vi "Outputs.vi"(0 "STEP in":T1, 5 "CORE":refnum<queue>, 7 "Mapping Buss":T9, 9 "STEP State":T8, 11 "error in (no error)":errorcluster, 12 "Variables State in":T6, 13 "HW CTRL Data":T7) -> (4 "STEP out":T1, 15 "error out":errorcluster)   [LabVIEW 2014, in "SeqLoop.lvlib"]
doc: "Gestiona las Salidas Digitales."
uses:
  TypeDefs/HW InOut MAP.ctl
  TypeDefs/STEP State.ctl
  APIs/Message Queue/Message Cluster.ctl
  TypeDefs/HW CTRL Data.ctl
  TypeDefs/HW Variables State.ctl
  TypeDefs/STEP.ctl
  TypeDefs/LogicParsedExpression.ctl
  Mimico Display/TypeDefs/Mimic Data.ctl
  Mimico Display/TypeDefs/BG Image.ctl
  Mimico Display/TypeDefs/mObject.ctl
  DO Monitoring Global Variables.vi
  APIs/Message Queue/Enqueue Message (Single).vi
  SeqLoop.lvlib
  APIs/Message Queue/WINFAS 2 Message Queue.lvlib
  Mimico Display/Mimico Display.lvlib
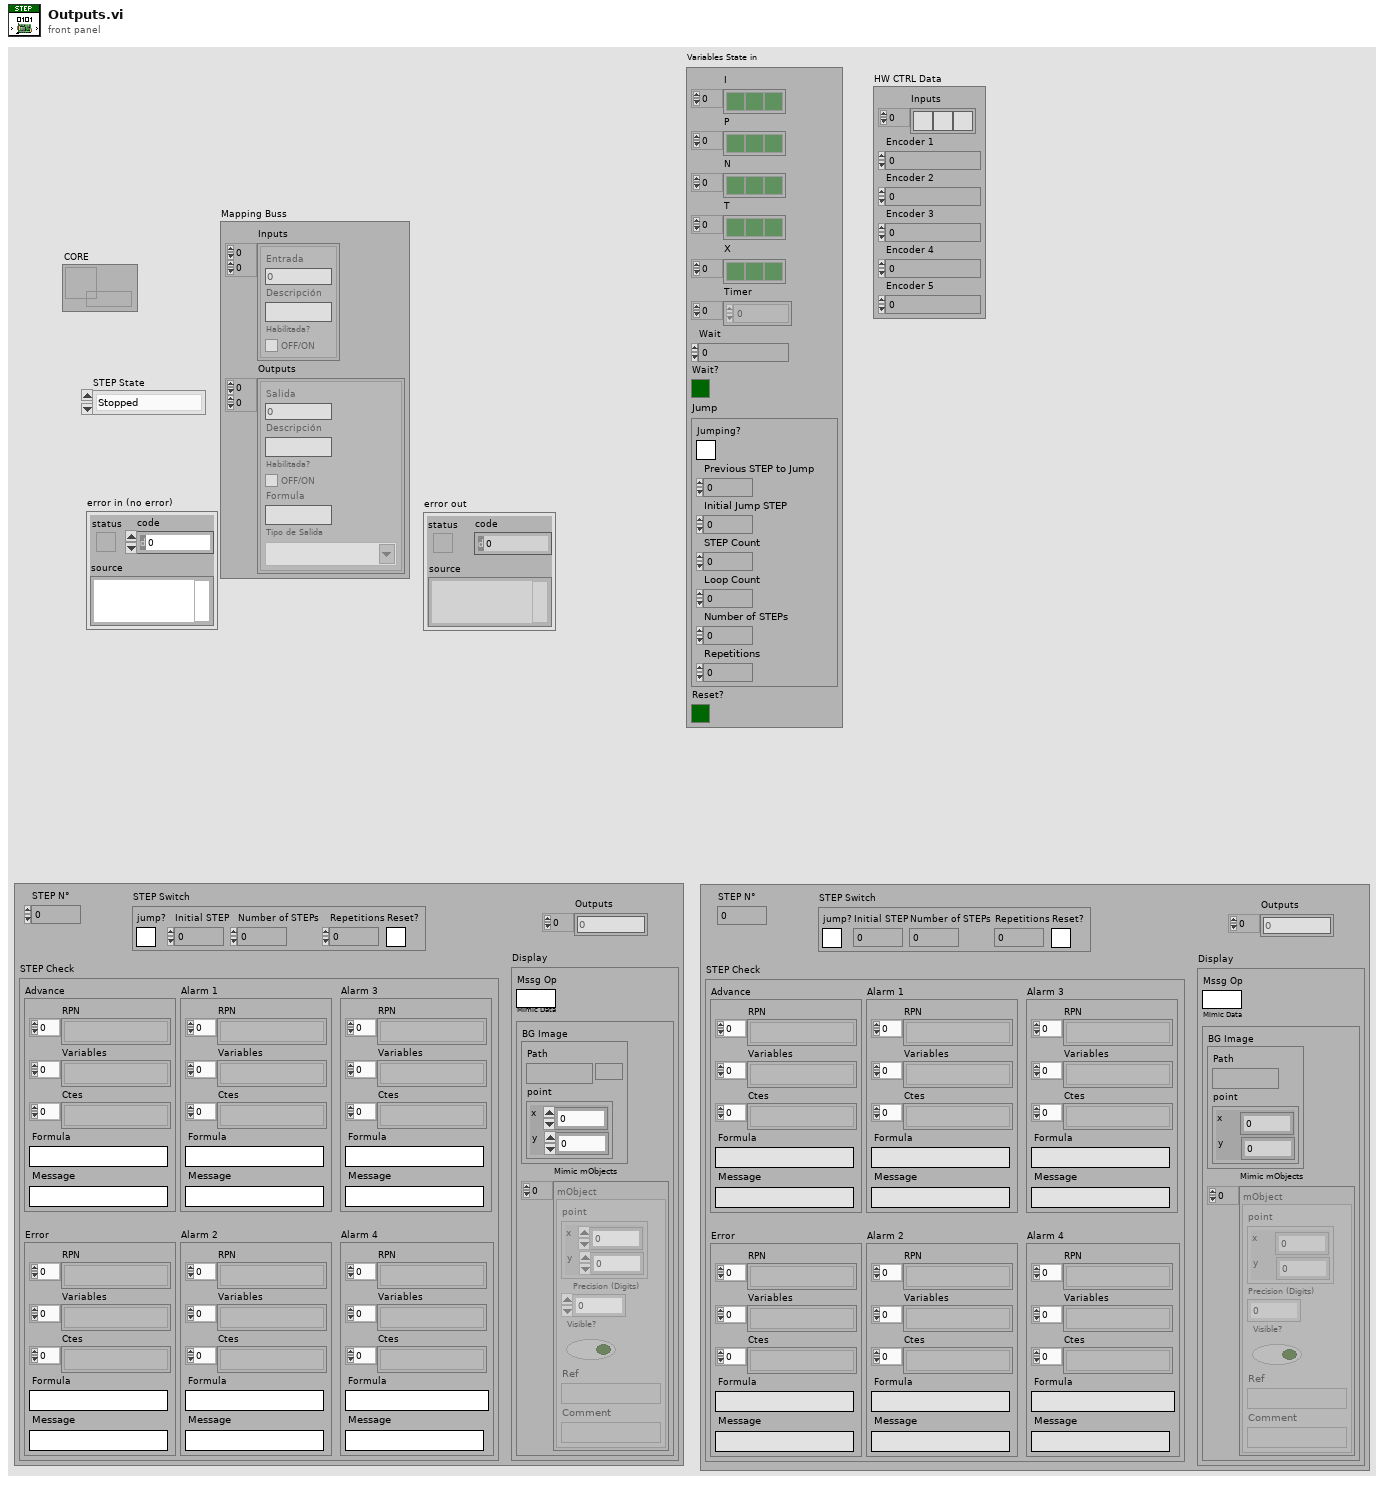
[diagram p1: front panel]
types:
  T1 = typedef "SeqLoop.lvlib/STEP.ctl" = cluster{"STEP N°":u32, "STEP Switch":cluster{"jump?":bool, "Initial STEP":u32, "Number of STEPs":u32, "Repetitions":u32, "Reset?":bool}, "Outputs":i32[], "STEP Check":cluster{"Advance":T2, "Error ":T2, "Alarm 1":T2, "Alarm 2":T2, "Alarm 3":T2, "Alarm 4":T2}, "Display":cluster{"Mssg Op":string, "Mimic Data":T3}}
  T2 = typedef "SeqLoop.lvlib/LogicParsedExpression.ctl" = cluster{"RPN ":string[], "Variables":string[], "Ctes":string[], "Formula":string, "Message":string}
  T3 = typedef "SeqLoop.lvlib/Mimico Display.lvlib/Mimic Data.ctl" = cluster{"BG Image":T4, "Mimic mObjects":T5[]}
  T4 = typedef "SeqLoop.lvlib/Mimico Display.lvlib/BG Image.ctl" = cluster{"Path":path, "point":cluster{"x":i16, "y":i16}}
  T5 = typedef "SeqLoop.lvlib/Mimico Display.lvlib/mObject.ctl" = cluster{"point":cluster{"x":i16, "y":i16}, "Precision (Digits)":i32, "Visible?":bool, "Ref":string, "Comment":string}
  T6 = typedef "SeqLoop.lvlib/HW Variables State.ctl" = cluster{"I":bool[], "P":bool[], "N":bool[], "T":bool[], "X":bool[], "Timer":u32[], "Wait":u32, "Wait?":bool, "Jump":cluster{"Jumping?":bool, "Previous STEP to Jump":u32, "Initial Jump STEP":u32, "STEP Count":u32, "Loop Count":u32, "Number of STEPs":u32, "Repetitions":u32}, "Reset?":bool}
  T7 = typedef "SeqLoop.lvlib/HW CTRL Data.ctl" = cluster{"Inputs":bool[], "Encoder 1":sgl, "Encoder 2":sgl, "Encoder 3":sgl, "Encoder 4":sgl, "Encoder 5":sgl}
  T8 = typedef "SeqLoop.lvlib/STEP State.ctl" = enum16{"Stopped", "First Call", "Idle...", "Advance OK", "Alarm", "Output Security", "Error"}
  T9 = typedef "SeqLoop.lvlib/HW InOut MAP.ctl" = cluster{"Inputs":cluster{"Entrada":i32, "Descripción":string, "Habilitada?":bool}[][], "Outputs":cluster{"Salida":i32, "Descripción":string, "Habilitada?":bool, "Formula":string, "Tipo de Salida":string}[][]}
  T10 = cluster{"DO Out[0]":bool, "DO Out[1]":bool, "DO Out[2]":bool, "DO Out[3]":bool, "DO Out[4]":bool, "DO Out[5]":bool, "DO Out[6]":bool, "DO Out[7]":bool, "DO Out[8]":bool, "DO Out[9]":bool, "DO Out[10]":bool, "DO Out[11]":bool, "DO Out[12]":bool, "DO Out[13]":bool, "DO Out[14]":bool, "DO Out[15]":bool, "DO Out[16]":bool, "DO Out[17]":bool, "DO Out[18]":bool, "DO Out[19]":bool, "DO Out[20]":bool, "DO Out[21]":bool, "DO Out[22]":bool, "DO Out[23]":bool, "DO Out[24]":bool, "DO Out[25]":bool, "DO Out[26]":bool, "DO Out[27]":bool, "DO Out[28]":bool, "DO Out[29]":bool, "DO Out[30]":bool, "DO Out[31]":bool}
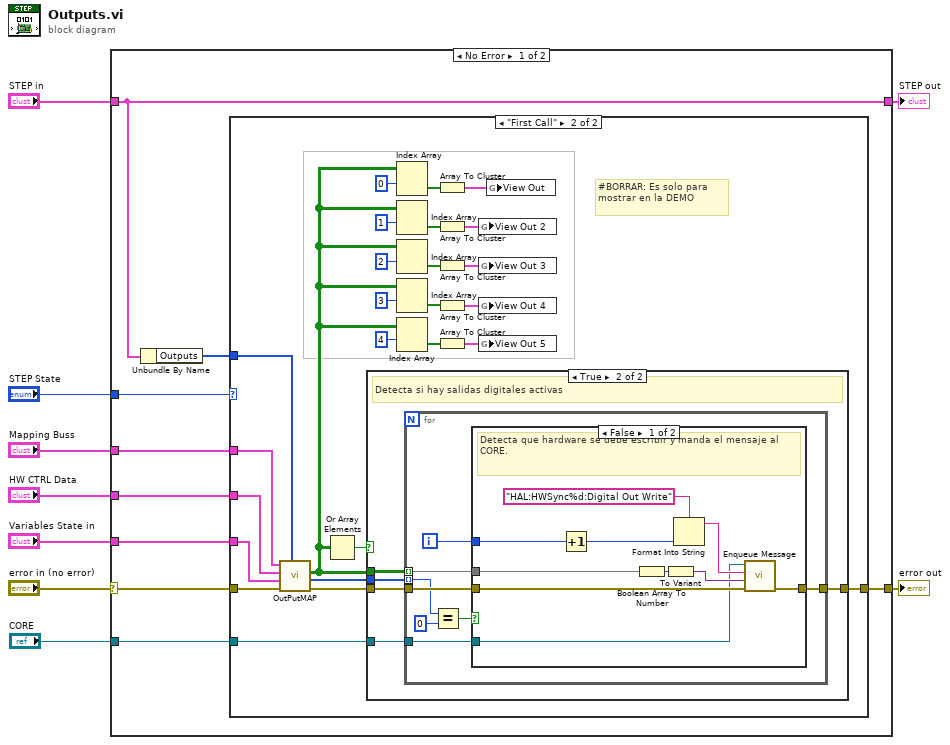
[diagram p0: block diagram]
diagram:
  n1 = case shown="No Error" "error in (no error)" {
    selector: "error in (no error)" -> [w14 w72]
    tunnel: [w12 w72] -> w8
    tunnel: [w16 w71] -> w1
    tunnel: "STEP in" -> [w16 w71]
    tunnel: "STEP State" -> [w18 _]
    tunnel: "Mapping Buss" -> [w17 _]
    tunnel: "CORE" -> [w13 _]
    tunnel: "HW CTRL Data" -> [w11 _]
    tunnel: "Variables State in" -> [w10 _]
    frame No Error {
      n2 = Unbundle By Name(w16) -> ("Outputs"=w15:i32[])
      n3 = case shown="\"First Call\"" w18 {
        tunnel: w17 -> [_ w44]
        tunnel: w15 -> [_ w22]
        tunnel: w14 -> [w19 w45]
        tunnel: [w19 w25] -> w12
        tunnel: w13 -> [_ w26]
        tunnel: w11 -> [_ w21]
        tunnel: w10 -> [_ w20]
        frame Default {
        }
        frame "First Call" {
          # "#BORRAR: Es solo para mostrar en la DEMO"
          n4 = call "OutPutMAP.vi"("Outputs"=w22, "error in (no error)"=w45, "Variables State in"=w20, "HW CTRL Data"=w21, "I/O Map In"=w44) -> ("error out"=w27:errorcluster, "DO Status"=w28:i32[], "DO Out"=w24:bool[][])  [unwired: 4 in]
          n5 = Or Array Elements(Boolean array=w24) -> (logical OR=w23:bool)
          n6 = case shown="True" w23 {
            tunnel: w28 -> [_ w51]
            tunnel: w27 -> [w46 w50]
            tunnel: w26 -> [_ w49]
            tunnel: [w46 w48] -> w25
            tunnel: w24 -> [_ w47]
            frame False {
              # "No se detecta escrituras de salidas digitales."
            }
            frame True {
              # "Detecta si hay salidas digitales activas"
              n7 = for {
                tunnel: w47 -> [w59] mode=indexing
                tunnel: w50 -> [w58]
                tunnel: [w57] -> w48
                tunnel: w49 -> [w56]
                tunnel: w51 -> [w53] mode=indexing
                i -> [w55]
                n8 = Equal?(x=w53, y=0 ("x")) -> (x = y?=w54:bool)
                n9 = case shown="False" w54 {
                  tunnel: w59 -> [w69 _]
                  tunnel: w58 -> [w66 w70]
                  tunnel: [w65 w70] -> w57
                  tunnel: w56 -> [w62 _]
                  tunnel: w55 -> [w61 _]
                  frame False {
                    # "Detecta que hardware se debe escribir y manda el mensaje al CORE."
                    n10 = Increment(x=w61) -> (x+1=w60:i32)
                    n11 = Boolean Array To Number(Boolean array=w69) -> (number=w68:u32)
                    n12 = To Variant(anything=w68) -> (Variant=w67:variant)
                    n13 = Format Into String(format string="HAL:HWSync%d:Digital Out Write" ("Message"), w60) -> (resulting string=w64:string)  [unwired: 2 in, 1 out]
                    n14 = call-poly "Enqueue Message.vi"("error in (no error)"=w66, "Message Data"=w67, "Message"=w64, "Message Queue"=w62) -> ("error out"=w65:errorcluster)  [unwired: 6 in, 1 out]
                  }
                  frame True {
                    # "No se detecta Hardware."
                  }
                }
              }
            }
          }
          n15 = Index Array(array=w24, index (row)=0) -> (element=w29:bool[])  [unwired: 1 in]
          n16 = Index Array(array=w24, index (row)=1) -> (element=w33:bool[])  [unwired: 1 in]
          n17 = Index Array(array=w24, index (row)=2) -> (element=w34:bool[])  [unwired: 1 in]
          n18 = Index Array(array=w24, index (row)=3) -> (element=w37:bool[])  [unwired: 1 in]
          n19 = Index Array(array=w24, index (row)=4) -> (element=w38:bool[])  [unwired: 1 in]
          n20 = Array To Cluster(array=w29) -> (cluster=w30:T10)
          n21 = Array To Cluster(array=w33) -> (cluster=w40:T10)
          n22 = Array To Cluster(array=w34) -> (cluster=w41:T10)
          n23 = Array To Cluster(array=w37) -> (cluster=w42:T10)
          n24 = Array To Cluster(array=w38) -> (cluster=w43:T10)
          n25 = global write "DO Monitoring Global Variables.vi" "View Out 2"(w40) -> ()
          n26 = global write "DO Monitoring Global Variables.vi" "View Out 3"(w41) -> ()
          n27 = global write "DO Monitoring Global Variables.vi" "View Out 4"(w42) -> ()
          n28 = global write "DO Monitoring Global Variables.vi" "View Out 5"(w43) -> ()
          n29 = global write "DO Monitoring Global Variables.vi" "View Out"(w30) -> ()
        }
      }
    }
    frame Error {
    }
  }
  "error out" <- w8
  "STEP out" <- w1
